vi "Read Data Config.vi"(8 "error in (no error)":errorcluster, 11 "ImagingExtractor in":refnum<class "ImagingExtractor.lvclass">) -> (0 "error out":errorcluster, 2 "Extracted Data Info":cluster{"Name":string, "Config":variant}[](array[cluster]), 3 "ImagingExtractor out":refnum<class "ImagingExtractor.lvclass">)   [LabVIEW 2014, in "ImagingExtractor.lvclass"]
uses:
  ImagingExtractor.lvclass
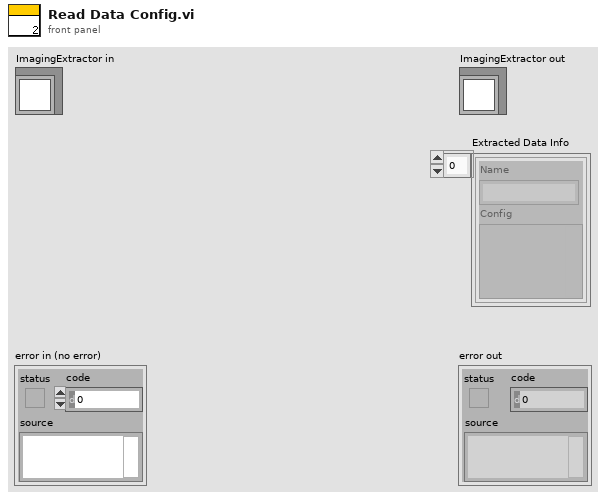
[diagram p1: front panel]
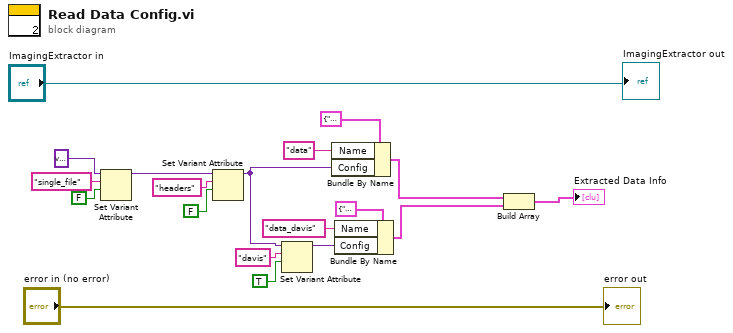
[diagram p0: block diagram]
diagram:
  n1 = Set Variant Attribute(Variant=variant ("variant"), name="single_file", value=FALSE ("Save to single file")) -> (Variant out=w14:variant)  [unwired: 1 in, 2 out]
  n2 = Set Variant Attribute(Variant=w14, name="headers", value=FALSE ("Save to single file")) -> (Variant out=w5:variant)  [unwired: 1 in, 2 out]
  n3 = Set Variant Attribute(Variant=w5, name="davis", value=TRUE ("Save to single file")) -> (Variant out=w4:variant)  [unwired: 1 in, 2 out]
  n4 = Bundle By Name(cluster=cluster{"Name":string, "Config":variant} {"Name"="", "Config"=variant} ("Cluster"), "Name"="data", "Config"=w5) -> (w15:cluster{"Name":string, "Config":variant})
  n5 = Bundle By Name(cluster=cluster{"Name":string, "Config":variant} {"Name"="", "Config"=variant} ("Cluster"), "Name"="data_davis", "Config"=w4) -> (w1:cluster{"Name":string, "Config":variant})
  n6 = Build Array(w15, w1) -> (→"Extracted Data Info":cluster{"Name":string, "Config":variant}[])
  "error out" <- "error in (no error)"
  "ImagingExtractor out" <- "ImagingExtractor in"
